vi "generateAxisString.vi"(11 "Input":T1) -> (3 "axis string":string)   [LabVIEW 2018]
uses:
  pgfPlotAxis_t.ctl
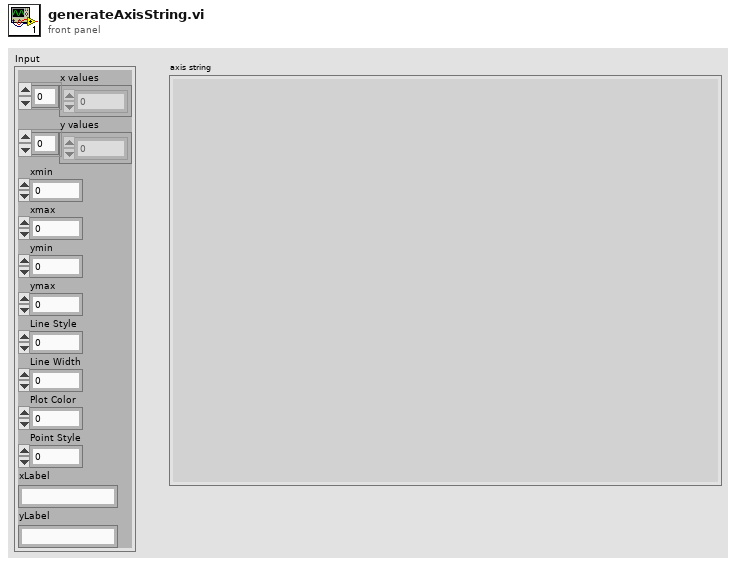
[diagram p1: front panel]
types:
  T1 = typedef "pgfPlotAxis_t.ctl" = cluster{"x values":dbl[], "y values":dbl[], "xmin":dbl, "xmax":dbl, "ymin":dbl, "ymax":dbl, "Line Style":u8, "Line Width":u8, "Plot Color":u32, "Point Style":u8, "xLabel":string, "yLabel":string}
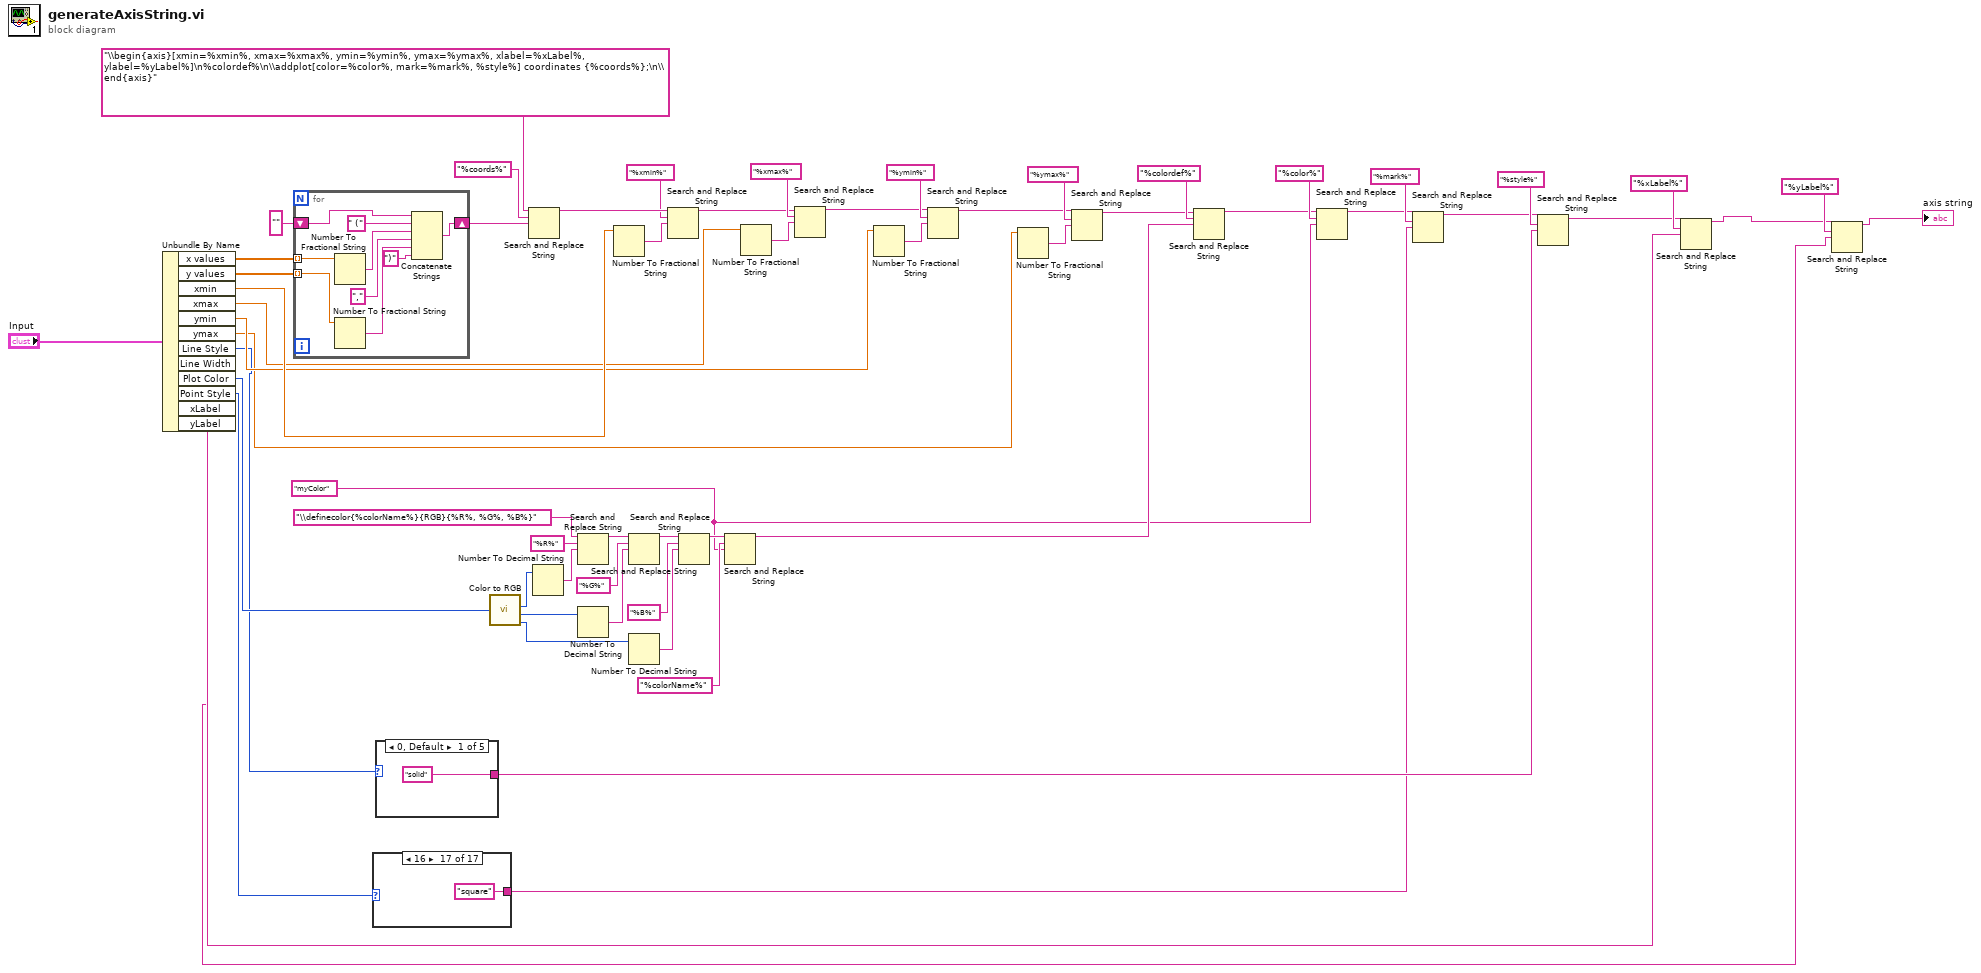
[diagram p0: block diagram]
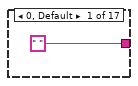
[diagram p2: hidden frame]
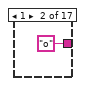
[diagram p3: hidden frame]
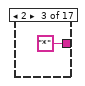
[diagram p4: hidden frame]
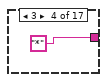
[diagram p5: hidden frame]
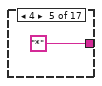
[diagram p6: hidden frame]
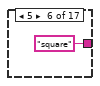
[diagram p7: hidden frame]
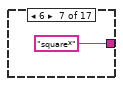
[diagram p8: hidden frame]
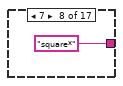
[diagram p9: hidden frame]
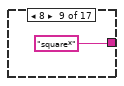
[diagram p10: hidden frame]
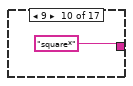
[diagram p11: hidden frame]
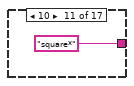
[diagram p12: hidden frame]
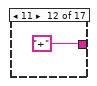
[diagram p13: hidden frame]
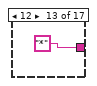
[diagram p14: hidden frame]
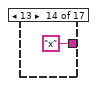
[diagram p15: hidden frame]
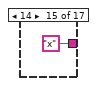
[diagram p16: hidden frame]
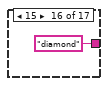
[diagram p17: hidden frame]
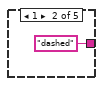
[diagram p18: hidden frame]
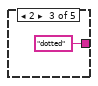
[diagram p19: hidden frame]
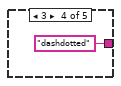
[diagram p20: hidden frame]
diagram:
  w14 = "myColor" ("replace string (\"\")")
  n1 = Unbundle By Name("Input") -> ("x values"=w57:dbl[], "y values"=w58:dbl[], "xmin"=w49:dbl, "xmax"=w39:dbl, "ymin"=w38:dbl, "ymax"=w37:dbl, "Line Style"=w13:u8, "Plot Color"=w30:u32, "Point Style"=w9:u8, "xLabel"=w2:string, "yLabel"=w1:string)  [unwired: 1 out]
  n2 = for {
    tunnel: w58 -> [w64] mode=indexing
    tunnel: w57 -> [w65] mode=indexing
    shift-right: [w67] -> w56
    shift-left: "" -> [w68]
    n3 = Number To Fractional String(number=w65) -> (F-format string=w63:string)  [unwired: 3 in]
    n4 = Number To Fractional String(number=w64) -> (F-format string=w61:string)  [unwired: 3 in]
    n5 = Concatenate Strings(w68, " (" ("string"), w63, "," ("string"), w61, ")" ("string")) -> (w67:string)
  }
  n6 = case shown="16" w9 {
    tunnel: [" " "o" "*" "*" "*" "square" "square*" "square*" "square*" "square*" "square*" "+" "*" "x" "x" "diamond" "square"] -> w8
    frame 0, Default {
    }
    frame 1 {
    }
    frame 2 {
    }
    frame 3 {
    }
    frame 4 {
    }
    frame 5 {
    }
    frame 6 {
    }
    frame 7 {
    }
    frame 8 {
    }
    frame 9 {
    }
    frame 10 {
    }
    frame 11 {
    }
    frame 12 {
    }
    frame 13 {
    }
    frame 14 {
    }
    frame 15 {
    }
    frame 16 {
    }
  }
  n7 = case shown="0, Default" w13 {
    tunnel: ["solid" "dashed" "dotted" "dashdotted" "dashdotdotted"] -> w10
    frame 0, Default {
    }
    frame 1 {
    }
    frame 2 {
    }
    frame 3 {
    }
    frame 4 {
    }
  }
  n8 = call <vilib>:"Color to RGB.vi"("Color"=w30) -> ("R"=w21:u8, "G"=w20:u8, "B"=w19:u8)  [unwired: 1 out]
  n9 = Search and Replace String(input string="\\begin{axis}[xmin=%xmin%, xmax=%xmax%, ymin=%ymin%, ymax=%ymax%, xlabel=%xLabel%, ylabel=%yLabel%]\n%colordef%\n\\addplot[color=%color%, mark=%mark%, %style%] coordinates {%coords%};\n\\end{axis}", search string="%coords%", replace string=w56) -> (result string=w52:string)  [unwired: 5 in, 3 out]
  n10 = Number To Decimal String(number=w21) -> (decimal integer string=w28:string)  [unwired: 1 in]
  n11 = Search and Replace String(input string="\\definecolor{%colorName%}{RGB}{%R%, %G%, %B%}", search string="%R%", replace string=w28) -> (result string=w23:string)  [unwired: 5 in, 3 out]
  n12 = Number To Decimal String(number=w20) -> (decimal integer string=w27:string)  [unwired: 1 in]
  n13 = Number To Fractional String(number=w49) -> (F-format string=w50:string)  [unwired: 3 in]
  n14 = Search and Replace String(input string=w23, search string="%G%", replace string=w27) -> (result string=w22:string)  [unwired: 5 in, 3 out]
  n15 = Number To Decimal String(number=w19) -> (decimal integer string=w24:string)  [unwired: 1 in]
  n16 = Search and Replace String(input string=w52, search string="%xmin%", replace string=w50) -> (result string=w42:string)  [unwired: 5 in, 3 out]
  n17 = Search and Replace String(input string=w22, search string="%B%", replace string=w24) -> (result string=w17:string)  [unwired: 5 in, 3 out]
  n18 = Search and Replace String(input string=w17, search string="%colorName%", replace string=w14) -> (result string=w16:string)  [unwired: 5 in, 3 out]
  n19 = Number To Fractional String(number=w39) -> (F-format string=w48:string)  [unwired: 3 in]
  n20 = Search and Replace String(input string=w42, search string="%xmax%", replace string=w48) -> (result string=w41:string)  [unwired: 5 in, 3 out]
  n21 = Number To Fractional String(number=w38) -> (F-format string=w45:string)  [unwired: 3 in]
  n22 = Search and Replace String(input string=w41, search string="%ymin%", replace string=w45) -> (result string=w40:string)  [unwired: 5 in, 3 out]
  n23 = Number To Fractional String(number=w37) -> (F-format string=w44:string)  [unwired: 3 in]
  n24 = Search and Replace String(input string=w40, search string="%ymax%", replace string=w44) -> (result string=w33:string)  [unwired: 5 in, 3 out]
  n25 = Search and Replace String(input string=w33, search string="%colordef%", replace string=w16) -> (result string=w32:string)  [unwired: 5 in, 3 out]
  n26 = Search and Replace String(input string=w32, search string="%color%", replace string=w14) -> (result string=w31:string)  [unwired: 5 in, 3 out]
  n27 = Search and Replace String(input string=w31, search string="%mark%", replace string=w8) -> (result string=w11:string)  [unwired: 5 in, 3 out]
  n28 = Search and Replace String(input string=w11, search string="%style%", replace string=w10) -> (result string=w5:string)  [unwired: 5 in, 3 out]
  n29 = Search and Replace String(input string=w5, search string="%xLabel%", replace string=w2) -> (result string=w4:string)  [unwired: 5 in, 3 out]
  n30 = Search and Replace String(input string=w4, search string="%yLabel%", replace string=w1) -> (result string=→"axis string":string)  [unwired: 5 in, 3 out]
